vi "Deg_Rad.vi"(8 "Rad":dbl, 11 "Deg":dbl) -> (0 "Deg":dbl, 3 "Rad":dbl)   [LabVIEW 2014]
doc: "弧度与角度转换"
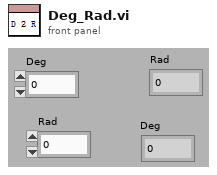
[diagram p1: front panel]
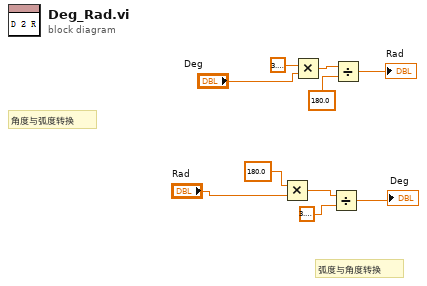
[diagram p0: block diagram]
diagram:
  # "弧度与角度转换"
  # "角度与弧度转换"
  n1 = Multiply(x=180.0 ("y"), y="Rad") -> (x*y=w2:dbl)
  n2 = Multiply(x=3.141592653589793, y="Deg") -> (x*y=w9:dbl)
  n3 = Divide(x=w2, y=3.141592653589793) -> (x/y=→"Deg":dbl)
  n4 = Divide(x=w9, y=180.0) -> (x/y=→"Rad":dbl)
